vi "Configure ECAT Generic Slave.vi"(8 "error in":errorcluster, 10 "Distributed Clock":bool, 11 "IOV ref":refnum<k21>) -> (0 "error out":errorcluster, 2 "Distributed Clock out":bool, 3 "IOV ref out":refnum<k21>)   [LabVIEW 2020, in "SEECD Engine.lvlib"]
uses:
  SEECD Engine.lvlib
  <resource>/objmgr/IndComECAT.rc
  <vilib>/NI VeriStand/Custom Device Tools/Custom Device Utility Library/Custom Device Utility Library.lvlib
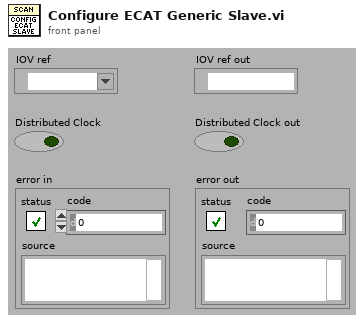
[diagram p1: front panel]
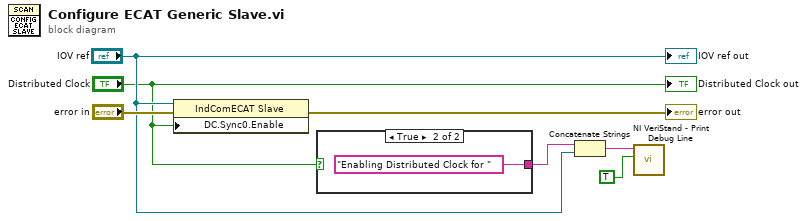
[diagram p0: block diagram]
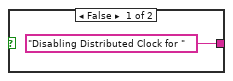
[diagram p2: hidden frame]
diagram:
  n1 = property class="IndComECAT Slave"(reference="IOV ref", error in="error in", "DC.Sync0.Enable"="Distributed Clock") -> (error out=→"error out":errorcluster)  [unwired: 1 out]
  n2 = case shown="True" "Distributed Clock" {
    tunnel: ["Disabling Distributed Clock for " "Enabling Distributed Clock for "] -> w2
    frame False {
    }
    frame True {
    }
  }
  n3 = Concatenate Strings(w2, "IOV ref") -> (w4:string)
  n4 = call <vilib>:"NI VeriStand - Print Debug Line.vi"("Add to log file? (F)"=TRUE, "Message"=w4) -> ()  [unwired: 9 in, 1 out]
  "IOV ref out" <- "IOV ref"
  "Distributed Clock out" <- "Distributed Clock"
